vi "_interfacebrowser build tree table in CSM-VI mode.vi"(6 "Config Path":path, 8 "Error in":errorcluster caption="Error in (no error)") -> (0 "Error out":errorcluster, 2 "Type":string[](array[string]), 3 "Tree Table":string[][](array[string]))   [LabVIEW 2017]
uses:
  _csmHelper/API with lvcsm Support/CSM-Helper API with lvcsm Support.lvlib
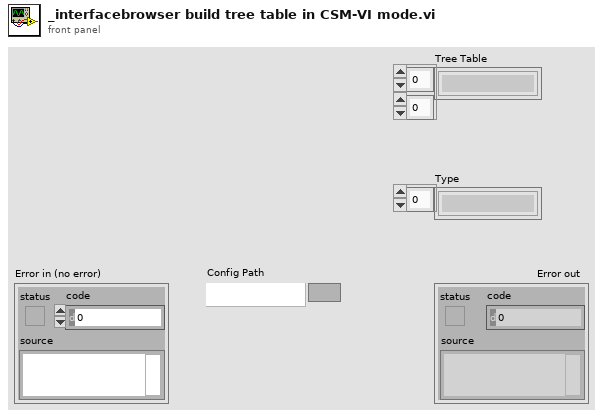
[diagram p1: front panel]
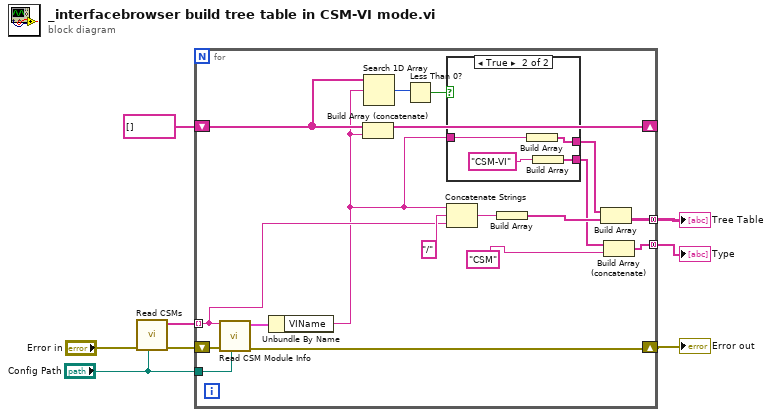
[diagram p0: block diagram]
diagram:
  n1 = call "Read CSMs.vi"("Config Path"="Config Path", "Error in"="Error in") -> ("Error out"=w5:errorcluster, "Array"=w8:string[])  [unwired: 8 in]
  n2 = for {
    tunnel: w8 -> [w24] mode=indexing
    tunnel: [w21] -> w2 mode=concatenating
    shift-right: [w20] -> _
    shift-left: string[] [] ("Delimiter") -> [w19]
    tunnel: [w13] -> w1 mode=concatenating
    tunnel: "Config Path" -> [w10]
    shift-right: [w9] -> w3
    shift-left: w5 -> [w11]
    n3 = call "Read CSM Module Info.vi"("Config Path"=w10, "error in (no error)"=w11, "CSM Name"=w24) -> ("error out"=w9:errorcluster, "Cluster"=w26:cluster{"VIName":string})  [unwired: 7 in]
    n4 = Unbundle By Name(w26) -> ("VIName"=w16:string)
    n5 = Build Array (concatenate)(w19, w16) -> (w20:string[])
    n6 = Search 1D Array(1D array=w19, element=w16) -> (index of element=w18:i32)  [unwired: 1 in]
    n7 = Less Than 0?(x=w18) -> (x < 0?=w17:bool)
    n8 = case shown="True" w17 {
      tunnel: w16 -> [_ w30]
      tunnel: [_ w29] -> w15
      tunnel: [_ w27] -> w14
      frame False {
      }
      frame True {
        n9 = Build Array(w30) -> (w29:string[])
        n10 = Build Array("CSM-VI" ("Delimiter")) -> (w27:string[])
      }
    }
    n11 = Concatenate Strings(w16, "/" ("Delimiter"), w24) -> (w23:string)
    n12 = Build Array(w23) -> (w22:string[])
    n13 = Build Array(w15, w22) -> (w21:string[][])
    n14 = Build Array (concatenate)(w14, "CSM" ("Delimiter")) -> (w13:string[])
  }
  "Type" <- w1
  "Tree Table" <- w2
  "Error out" <- w3
